vi "eMbot_EMG_viewer fun with shift registers.vi"() -> ()   [LabVIEW 2011]
uses:
  <vilib>/Utility/file.llb/Read From Spreadsheet File (DBL).vi
  <vilib>/Analysis/3filter.llb/Butterworth Filter (DBL).vi
  <vilib>/Analysis/1siggen.llb/Ramp Pattern by Samples.vi
  <vilib>/Analysis/8numeric.llb/1D Numeric Integration.vi
  <vilib>/Utility/file.llb/Write To Spreadsheet File (string).vi
  <vilib>/Analysis/NI_AALBase.lvlib
  <vilib>/Analysis/NI_AAL_SigProc.lvlib
  <vilib>/Analysis/NI_AALPro.lvlib
panel:
  in  "Use MVC?":bool
  in  "Data to Read":i32=-1
  in  "Side":u16(ring) items=["Right", "Left"]
  in  "Cycle-by-Cycle":bool=TRUE
  in  "Averaged Bins":bool=TRUE
  in  "Ensemble Averages":bool=TRUE
  in  "Select Muscles to Save":i32[](listbox)=[0, 1, 2, 3, 4, 5, 6, 7]
  in  "Save":bool
  in  "low cutoff freq":dbl=2.0
  in  "high cutoff freq":dbl=10.0
  in  "sampling freq":dbl=1000.0
  in  "Max EMG File":string="MVC1.txt"
  in  "Data Directory":string="C:\\Users\\PM&R\\Desktop\\Desktop Items\\Peter\\Data\\eMbot Testing Data\\"
  in  "Window Size":i32=10
  in  "peaks/valleys":enum32{"Peaks", "Valleys"}(ring)
  in  "Save Folder Name":string="EMG Postprocess"
  in  "Gait Event Channel":i32=18
  out "Locations":dbl[](array[numeric])
  in  "Stop":bool
  out "EMG Max":dbl
  in  "Threshold %Max":dbl=0.5
  in  "Shift Ensemble":i32
  out "RAW EMG":dbl[](graph)
  in  "Subject ID":string
  in  "Trial":i32
  out "Ensemble Average SD":dbl[](graph)
  out "Maximum EMG":dbl[](graph)
  out "Gait Event detection":cluster{"Ramp Pattern":dbl[], dbl[]}[](graph)
  in  "Muscle":i32
  out "Ensemble Average EMG":dbl[](graph)
  out "Spectrum Plot":cluster{dbl, "df":dbl, dbl[]}(graph)={0.0, "df"=0.5, []}
  out "Linear Envelope  EMG":dbl[](graph)
  out "Raw Gait Event Detection":dbl[](graph)
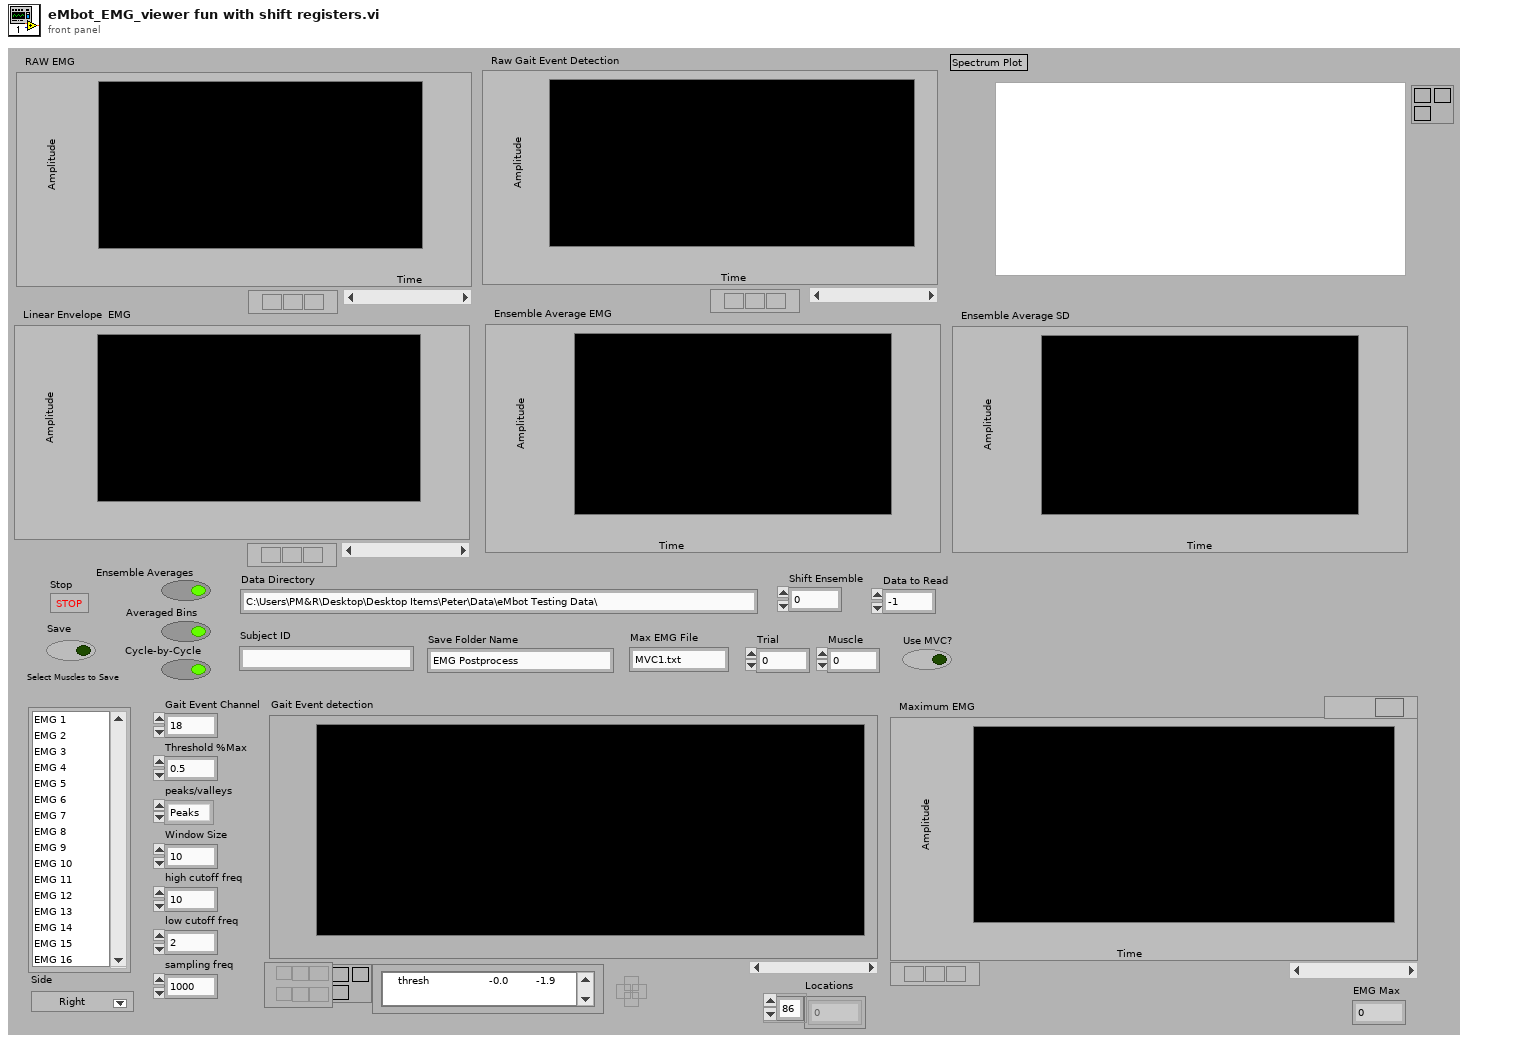
[diagram p1: front panel]
types:
  T1 = enum32{"Trapezoidal Rule", "Simpson's Rule", "Simpson's 3/8 Rule", "Bode Rule"}
  T2 = enum32{"Lowpass", "Highpass", "Bandpass", "Bandstop"}
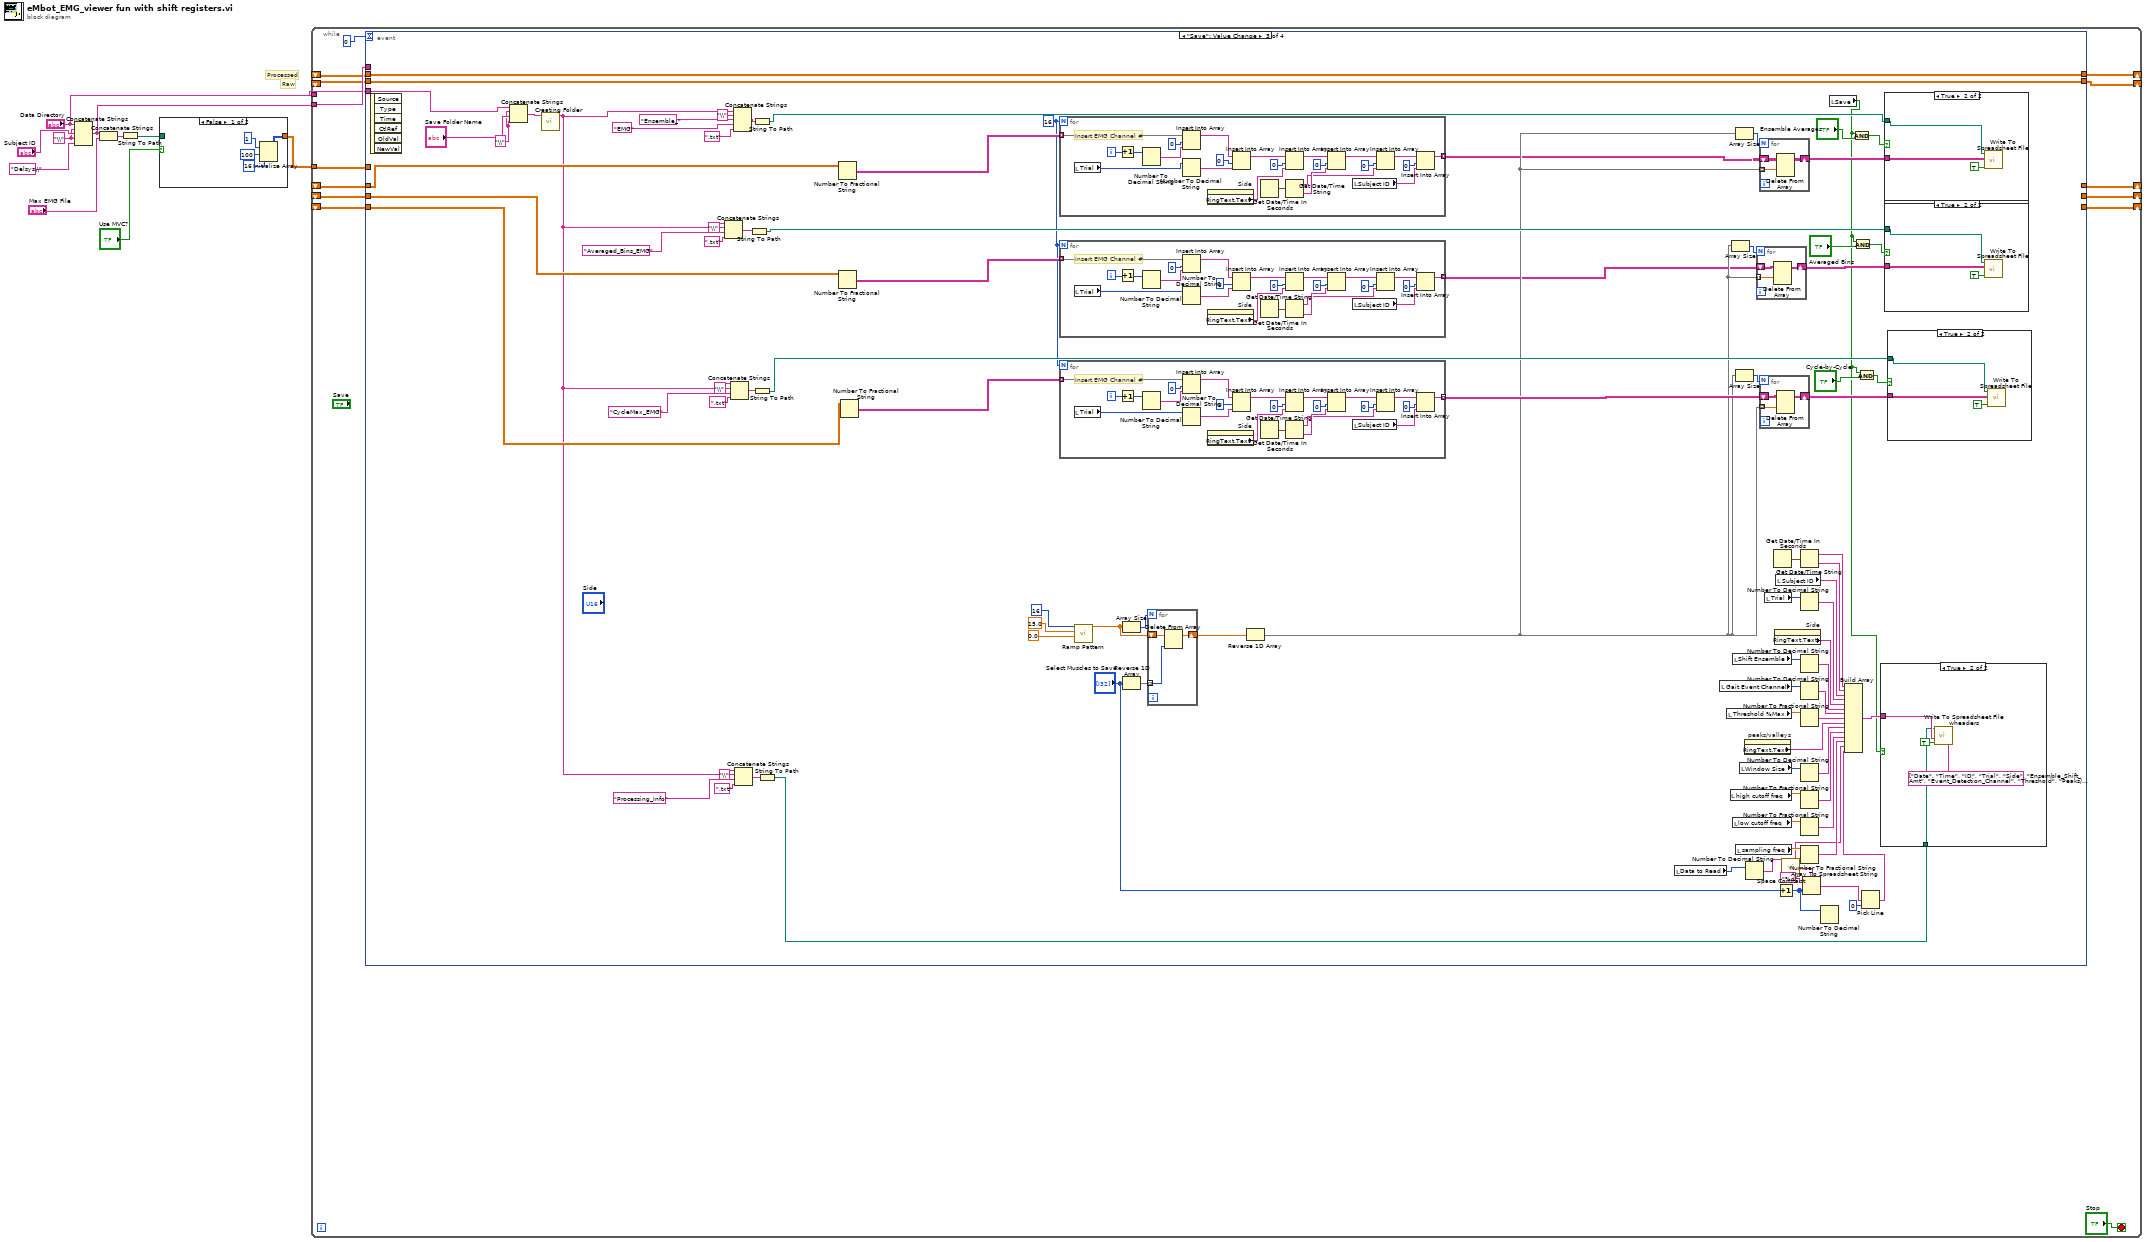
[diagram p0: block diagram]
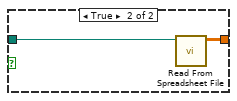
[diagram p2: hidden frame]
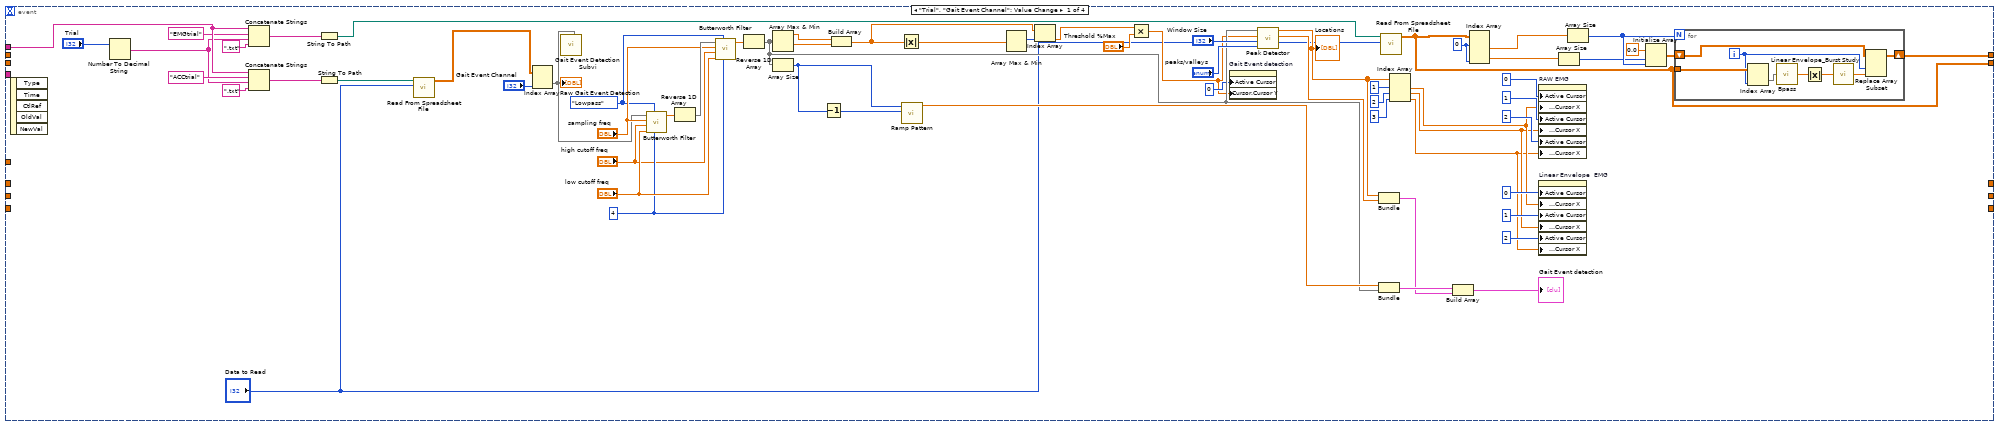
[diagram p3: hidden frame]
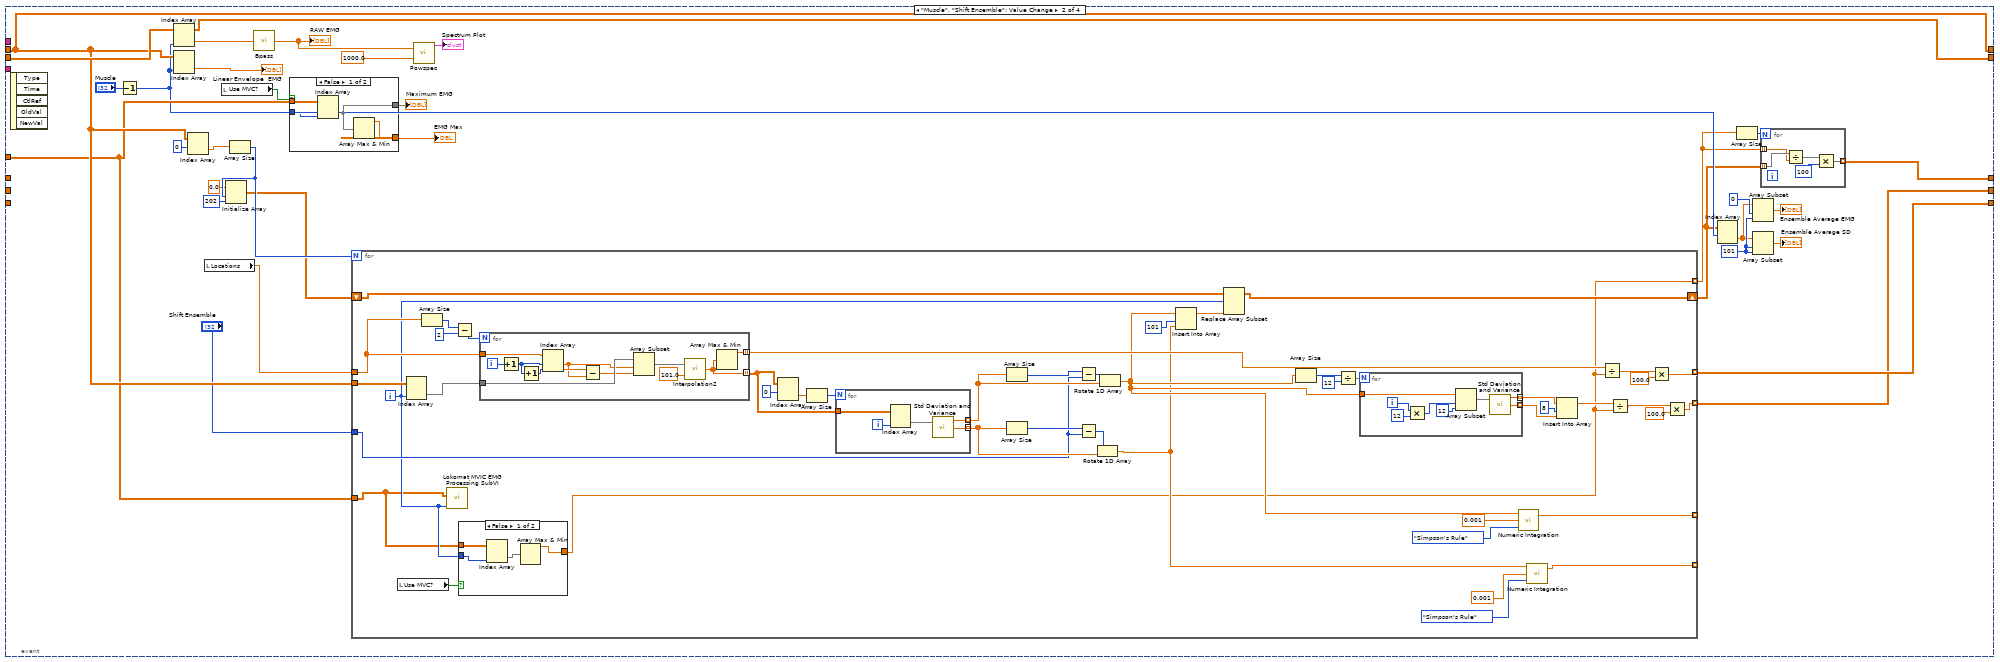
[diagram p4: hidden frame]
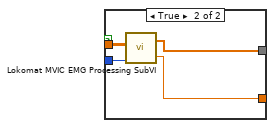
[diagram p5: hidden frame]
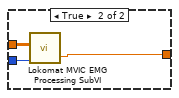
[diagram p6: hidden frame]
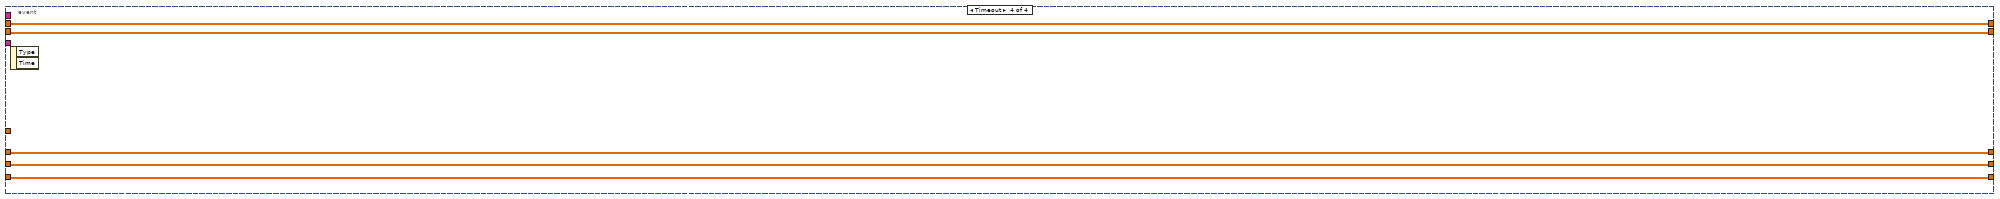
[diagram p11: hidden frame]
diagram:
  w3 = "\\" ("string")
  # "Raw"
  # "Processed"
  n1 = Concatenate Strings("Data Directory", w3, "Subject ID", w3, "Delsys\\" ("string")) -> (w5:string)
  n2 = Concatenate Strings(w5, "Max EMG File") -> (w8:string)
  n3 = String To Path(string=w8) -> (path=w9:path)
  n4 = case shown="False" "Use MVC?" {
    tunnel: w9 -> [_ w16]
    tunnel: [w13 w15] -> w4
    frame False {
      n5 = Initialize Array(1, 100 ("dimension size"), 16 ("dimension size")) -> (w13:i32[][])
    }
    frame True {
      n6 = call-poly <vilib>:"Read From Spreadsheet File.vi"("file path (dialog if empty)"=w16) -> ("all rows"=w15:dbl[][])  [unwired: 6 in, 4 out]
    }
  }
  n7 = while {
    tunnel: w5 -> [w30]
    tunnel: w4 -> [w28]
    shift-right: [w27] -> _
    shift-left: _ -> [w26]
    shift-right: [w25] -> _
    shift-left: _ -> [w24]
    shift-right: [w23] -> _
    shift-left: _ -> [w22]
    shift-right: [w21] -> _
    shift-left: _ -> [w20]
    shift-right: [w19] -> _
    shift-left: _ -> [w18]
    tunnel: "Data Directory" -> [w17]
    stop <- "Stop" stop-if-true
    n8 = event shown="[2] \"Save\": Value Change" {
      selector: _ -> [_ _ _ _]
      dyn-events: _ -> [_ _ _ _]
      timeout: 0 -> [_ _ _ _]
      tunnel: w30 -> [w62 _ _ _]
      tunnel: w28 -> [_ w114 _ _]
      tunnel: [_ w131 _ w413] -> w19
      tunnel: [w39 w126 w318 w417] -> w27
      tunnel: w26 -> [_ w126 w318 w417]
      tunnel: [w40 w127 w317 w416] -> w25
      tunnel: w24 -> [_ w127 w317 w416]
      tunnel: [_ w107 _ w415] -> w23
      tunnel: w22 -> [_ _ w305 w415]
      tunnel: [_ w106 _ w414] -> w21
      tunnel: w20 -> [_ _ w301 w414]
      tunnel: w18 -> [_ _ w293 w413]
      tunnel: w17 -> [_ _ w297 _]
      event "Trial", "Gait Event Channel": Value Change {
        w37 = 0 ("index (row)")
        w81 = T2."Lowpass" ("filter type")
        w82 = 4 ("order")
        n9 = event-data() -> ()  [unwired: 1 in, 5 out]
        n10 = Number To Decimal String(number="Trial") -> (decimal integer string=w56:string)  [unwired: 1 in]
        n11 = Concatenate Strings(w62, "EMGtrial" ("string"), w56, ".txt" ("string")) -> (w61:string)
        n12 = Concatenate Strings(w62, "ACCtrial" ("string"), w56, ".txt" ("string")) -> (w54:string)
        n13 = String To Path(string=w61) -> (path=w60:path)
        n14 = String To Path(string=w54) -> (path=w53:path)
        n15 = call-poly <vilib>:"Read From Spreadsheet File.vi"("number of rows (all:-1)"="Data to Read", "file path (dialog if empty)"=w53) -> ("all rows"=w95:dbl[][])  [unwired: 5 in, 4 out]
        n16 = Index Array(array=w95, index (col)="Gait Event Channel") -> (element=w50:dbl[])  [unwired: 1 in]
        "Raw Gait Event Detection" <- w50
        n17 = call "Gait Event Detection Subvi.vi"("Array"=w50) -> ()  [unwired: 1 in, 10 out]
        n18 = call-poly <vilib>:"Butterworth Filter.vi"("order"=w82, "filter type"=w81, "low cutoff freq: fl"="low cutoff freq", "high cutoff freq: fh"="high cutoff freq", "sampling freq: fs"="sampling freq", "X"=w50) -> ("Filtered X"=w87:dbl[])  [unwired: 2 in, 1 out]
        n19 = Reverse 1D Array(array=w87) -> (reversed array=w86:dbl[])
        n20 = call-poly <vilib>:"Butterworth Filter.vi"("order"=w82, "filter type"=w81, "low cutoff freq: fl"="low cutoff freq", "high cutoff freq: fh"="high cutoff freq", "sampling freq: fs"="sampling freq", "X"=w86) -> ("Filtered X"=w83:dbl[])  [unwired: 2 in, 1 out]
        n21 = Reverse 1D Array(array=w83) -> (reversed array=w64:dbl[])
        n22 = Array Max & Min(array=w64) -> (max value=w47:dbl, min value=w46:dbl)  [unwired: 2 out]
        n23 = Array Size(array=w64) -> (size(s)=w75:i32)
        n24 = Decrement(x=w75) -> (x-1=w76:i32)
        n25 = Build Array(w47, w46) -> (w43:dbl[])
        n26 = Absolute Value(x=w43) -> (abs(x)=w45:dbl[])
        n27 = call-poly <vilib>:"Ramp Pattern.vi"("end"=w76, "samples"=w75) -> ("Ramp Pattern"=w77:dbl[])  [unwired: 8 in, 1 out]
        n28 = Array Max & Min(array=w45) -> (max index (indices)=w42:i32)  [unwired: 3 out]
        n29 = Index Array(array=w43, index=w42) -> (element=w44:dbl)
        n30 = Multiply(x=w44, y="Threshold %Max") -> (x*y=w48:dbl)
        n31 = property on="Gait Event detection" class="XYGraph (strict)"("Active Cursor"=u32 0, "Cursor.Cursor Y"=w48) -> ()  [unwired: 2 in, 2 out]
        n32 = call <vilib>:"Peak Detector.vi"("peaks/valleys"="peaks/valleys", "width"="Window Size", "threshold"=w48, "X"=w64) -> ("Amplitudes"=w73:dbl[], "Locations"=w51:dbl[])  [unwired: 3 in, 3 out]
        "Locations" <- w51
        n33 = Bundle("Locations"=w51, "Amplitudes"=w73) -> (w72:cluster{"Locations":dbl[], "Amplitudes":dbl[]})  [unwired: 1 in]
        n34 = Bundle("Ramp Pattern"=w77, w64) -> (w74:cluster{"Ramp Pattern":dbl[], dbl[]})  [unwired: 1 in]
        n35 = call-poly <vilib>:"Read From Spreadsheet File.vi"("number of rows (all:-1)"="Data to Read", "file path (dialog if empty)"=w60) -> ("all rows"=w40:dbl[][])  [unwired: 5 in, 4 out]
        n36 = Index Array(array=w51, index #1=1 ("index"), index #2=2 ("index"), index #3=3 ("index")) -> (element #1=w67:dbl, element #2=w66:dbl, element #3=w65:dbl)
        n37 = Build Array(w74, w72) -> (→"Gait Event detection":cluster{"Locations":dbl[], "Amplitudes":dbl[]}[])
        n38 = Index Array(array=w40, index (row) #1=w37, index (col) #2=w37) -> (element #1=w41:dbl[], element #2=w36:dbl[])  [unwired: 2 in]
        n39 = property on="RAW EMG" class="WFGraph (strict)"("Active Cursor"=u32 0, "Cursor.Cursor Position:Cursor X"=w67, "Active Cursor"=u32 1, "Cursor.Cursor Position:Cursor X"=w66, "Active Cursor"=u32 2, "Cursor.Cursor Position:Cursor X"=w65) -> ()  [unwired: 2 in, 2 out]
        n40 = property on="Linear Envelope  EMG" class="WFGraph (strict)"("Active Cursor"=u32 0, "Cursor.Cursor Position:Cursor X"=w67, "Active Cursor"=u32 1, "Cursor.Cursor Position:Cursor X"=w66, "Active Cursor"=u32 2, "Cursor.Cursor Position:Cursor X"=w65) -> ()  [unwired: 2 in, 2 out]
        n41 = Array Size(array=w36) -> (size(s)=w35:i32)
        n42 = Array Size(array=w41) -> (size(s)=w38:i32)
        n43 = Initialize Array(0.0 ("element"), w35, w38) -> (w34:dbl[][])
        n44 = for {
          N: w38 -> [_]
          tunnel: w40 -> [w101]
          shift-right: [w96] -> w39
          shift-left: w34 -> [w98]
          i -> [w97]
          n45 = Index Array(array=w101, index (col)=w97) -> (element=w100:dbl[])  [unwired: 1 in]
          n46 = call "Bpass.vi"("Input Array"=w100) -> ("Output Array"=w102:dbl[])
          n47 = Absolute Value(x=w102) -> (abs(x)=w103:dbl[])
          n48 = call "Linear Envelope_Burst Study.vi"("Signals"=w103) -> ("Filtered Signals"=w99:dbl[])
          n49 = Replace Array Subset(array=w98, new element=w99, index (col)=w97) -> (w96:dbl[][])  [unwired: 1 in]
        }
      }
      event "Muscle", "Shift Ensemble": Value Change {
        w116 = 101 ("length")
        n50 = event-data() -> ()  [unwired: 1 in, 5 out]
        n51 = Decrement(x="Muscle") -> (x-1=w113:i32)
        n52 = Index Array(array=w127, index (col)=w113) -> (element=w130:dbl[])  [unwired: 1 in]
        n53 = Index Array(array=w126, index (col)=w113) -> (element=→"Linear Envelope  EMG":dbl[])  [unwired: 1 in]
        n54 = Index Array(array=w126, index (row)=0) -> (element=w124:dbl[])  [unwired: 1 in]
        n55 = local read "Locations"() -> (w132:dbl[])
        n56 = local read "Use MVC?"() -> (w104:bool)
        n57 = Array Size(array=w124) -> (size(s)=w123:i32)
        n58 = Initialize Array(0.0 ("element"), w123, 202 ("dimension size")) -> (w121:dbl[][])
        n59 = call "Bpass.vi"("Input Array"=w130) -> ("Output Array"=w129:dbl[])
        "RAW EMG" <- w129
        n60 = case shown="False" w104 {
          tunnel: w114 -> [w139 w143]
          tunnel: w113 -> [w138 w142]
          tunnel: [w137 w141] -> w112
          tunnel: [w136 w140] -> w111
          frame False {
            n61 = Index Array(array=w139, index (col)=w138) -> (element=w137:dbl[])  [unwired: 1 in]
            n62 = Array Max & Min(array=w137) -> (max value=w136:dbl)  [unwired: 3 out]
          }
          frame True {
            n63 = call "Lokomat MVIC EMG Processing SubVI.vi"("EMG Channel"=w142, "Input Array"=w143) -> ("EMG Max"=w140:dbl, "EMG"=w141:dbl[])  [unwired: 2 in]
          }
        }
        "Maximum EMG" <- w112
        "EMG Max" <- w111
        n64 = for {
          N: w123 -> [_]
          tunnel: w126 -> [w166]
          tunnel: w132 -> [w195]
          tunnel: [w172] -> w131 mode=indexing
          shift-right: [w158] -> w110
          shift-left: w121 -> [w161]
          tunnel: [w160] -> _ mode=indexing
          tunnel: [w159] -> _ mode=indexing
          tunnel: w114 -> [w150]
          tunnel: [w149] -> w108 mode=indexing
          tunnel: [w155] -> w106 mode=indexing
          tunnel: "Shift Ensemble" -> [w153]
          i -> [w151]
          n65 = local read "Use MVC?"() -> (w152:bool)
          n66 = Index Array(array=w166, index (col)=w151) -> (element=w165:dbl[])  [unwired: 1 in]
          n67 = Array Size(array=w195) -> (size(s)=w174:i32)
          n68 = call "Lokomat MVIC EMG Processing SubVI.vi"("EMG Channel"=w151, "Input Array"=w150) -> ()  [unwired: 2 in, 2 out]
          n69 = Subtract(x=w174, y=2) -> (x-y=w185:i32)
          n70 = case shown="False" w152 {
            tunnel: w150 -> [w199 w202]
            tunnel: w151 -> [w198 w201]
            tunnel: [w196 w200] -> w149
            frame False {
              n71 = Index Array(array=w199, index (col)=w198) -> (element=w197:dbl[])  [unwired: 1 in]
              n72 = Array Max & Min(array=w197) -> (max value=w196:dbl)  [unwired: 3 out]
            }
            frame True {
              n73 = call "Lokomat MVIC EMG Processing SubVI.vi"("EMG Channel"=w201, "Input Array"=w202) -> ("EMG Max"=w200:dbl)  [unwired: 2 in, 1 out]
            }
          }
          n74 = for {
            N: w185 -> [_]
            tunnel: w165 -> [w227]
            tunnel: w195 -> [w225]
            tunnel: [w217] -> w167 mode=indexing
            tunnel: [w216] -> w194 mode=indexing
            i -> [w226]
            n75 = Increment(x=w226) -> (x+1=w224:i32)
            n76 = Increment(x=w224) -> (x+1=w223:i32)
            n77 = Index Array(array=w225, index #1=w224, index #2=w223) -> (element #1=w218:dbl, element #2=w222:dbl)
            n78 = Subtract(x=w222, y=w218) -> (x-y=w219:dbl)
            n79 = Array Subset(array=w227, index=w218, length=w219) -> (w221:dbl[])
            n80 = call "Interpolation2.vi"("Normalize to # of Data Points"=101.0, "Original Array"=w221) -> ("Normalized Array"=w217:dbl[])
            n81 = Array Max & Min(array=w217) -> (max value=w216:dbl)  [unwired: 3 out]
          }
          n82 = Index Array(array=w167, index (row)=0) -> (element=w177:dbl[])  [unwired: 1 in]
          n83 = Array Size(array=w177) -> (size(s)=w178:i32)
          n84 = for {
            N: w178 -> [_]
            tunnel: w167 -> [w215]
            tunnel: [w212] -> w188 mode=indexing
            tunnel: [w211] -> w191 mode=indexing
            i -> [w214]
            n85 = Index Array(array=w215, index (col)=w214) -> (element=w213:dbl[])  [unwired: 1 in]
            n86 = call <vilib>:"Std Deviation and Variance.vi"("X"=w213) -> ("mean"=w212:dbl, "standard deviation"=w211:dbl)  [unwired: 1 in, 1 out]
          }
          n87 = Array Size(array=w188) -> (size(s)=w186:i32)
          n88 = Array Size(array=w191) -> (size(s)=w189:i32)
          n89 = Subtract(x=w186, y=w153) -> (x-y=w187:i32)
          n90 = Subtract(x=w189, y=w153) -> (x-y=w190:i32)
          n91 = Rotate 1D Array(1:w191, 2:w190) -> (0:w163:dbl[])
          n92 = Rotate 1D Array(1:w188, 2:w187) -> (0:w164:dbl[])
          n93 = Insert Into Array(array=w164, index=101, new element=w163) -> (w162:dbl[])
          n94 = Replace Array Subset(array=w161, new element=w162, index (row)=w151) -> (w158:dbl[][])  [unwired: 1 in]
          n95 = Array Size(array=w164) -> (size(s)=w180:i32)
          n96 = Divide(x=w180, y=12) -> (x/y=w179:dbl)
          n97 = for {
            N: w179 -> [_]
            tunnel: w164 -> [w210]
            tunnel: [w204] -> w182 mode=indexing
            tunnel: [w203] -> w184 mode=indexing
            i -> [w209]
            n98 = Multiply(x=w209, y=12) -> (x*y=w207:i32)
            n99 = Array Subset(array=w210, index=w207, length=12) -> (w205:dbl[])
            n100 = call <vilib>:"Std Deviation and Variance.vi"("X"=w205) -> ("mean"=w204:dbl, "standard deviation"=w203:dbl)  [unwired: 1 in, 1 out]
          }
          n101 = call-poly <vilib>:"Numeric Integration.vi"("integration method"=T1."Simpson's Rule", "dt"=0.001, "Input Array"=w164) -> ("result"=w160:dbl)  [unwired: 1 out]
          n102 = call-poly <vilib>:"Numeric Integration.vi"("integration method"=T1."Simpson's Rule", "dt"=0.001, "Input Array"=w163) -> ("result"=w159:dbl)  [unwired: 1 out]
          n103 = Insert Into Array(array=w182, index=8, new element=w184) -> (w157:dbl[])
          n104 = Divide(x=w194, y=w149) -> (x/y=w192:dbl[])
          n105 = Divide(x=w157, y=w149) -> (x/y=w154:dbl[])
          n106 = Multiply(x=w192, y=100.0) -> (x*y=w172:dbl[])
          n107 = Multiply(x=w154, y=100.0) -> (x*y=w155:dbl[])
        }
        n108 = call "Powspec.vi"("Emg input"=w129, "Sample rate"=sgl 1000.0) -> ("Spectrum Plot"=→"Spectrum Plot":cluster{dbl, "df":dbl, dbl[]})  [unwired: 5 out]
        n109 = Index Array(array=w110, index (row)=w113) -> (element=w115:dbl[])  [unwired: 1 in]
        n110 = Array Size(array=w108) -> (size(s)=w109:i32)
        n111 = Array Subset(array=w115, index=0, length=w116) -> (→"Ensemble Average EMG":dbl[])
        n112 = Array Subset(array=w115, index=w116, length=w116) -> (→"Ensemble Average SD":dbl[])
        n113 = for {
          N: w109 -> [_]
          tunnel: w108 -> [w147] mode=indexing
          tunnel: w110 -> [w148] mode=indexing
          tunnel: [w144] -> w107 mode=indexing
          n114 = Divide(x=w148, y=w147) -> (x/y=w146:dbl[])
          n115 = Multiply(x=w146, y=100) -> (x*y=w144:dbl[])
        }
      }
      event "Save": Value Change {
        w231 = 16
        w298 = "\\" ("string")
        n116 = event-data() -> ()  [unwired: 1 in, 6 out]
        n117 = Concatenate Strings(w297, w298, "Save Folder Name", w298) -> (w316:string)
        n118 = call "Creating Folder.vi"("Input String Path"=w316) -> ("Output String Path"=w254:string)  [unwired: 10 in]
        n119 = Concatenate Strings(w254, "\\" ("string"), "Averaged_Bins_EMG", ".txt" ("string")) -> (w308:string)
        n120 = Concatenate Strings(w254, "\\" ("string"), "CycleMax_EMG", ".txt" ("string")) -> (w313:string)
        n121 = Concatenate Strings(w254, "\\" ("string"), "Ensemble_" ("string"), "EMG", ".txt" ("string")) -> (w310:string)
        n122 = Concatenate Strings(w254, "\\" ("string"), "Processing_Info", ".txt" ("string")) -> (w256:string)
        n123 = String To Path(string=w308) -> (path=w302:path)
        n124 = String To Path(string=w310) -> (path=w306:path)
        n125 = String To Path(string=w313) -> (path=w299:path)
        n126 = String To Path(string=w256) -> (path=w253:path)
        n127 = Number To Fractional String(number=w305) -> (F-format string=w245:string[][])  [unwired: 3 in]
        n128 = Number To Fractional String(number=w301) -> (F-format string=w247:string[][])  [unwired: 3 in]
        n129 = Number To Fractional String(number=w293) -> (F-format string=w300:string[][])  [unwired: 3 in]
        n130 = for {
          N: w231 -> [_]
          tunnel: w245 -> [w343] mode=indexing
          tunnel: [w340] -> w244 mode=indexing
          i -> [w335]
          # "Insert EMG Channel #"
          n131 = local read "Trial"() -> (w336:i32)
          n132 = Increment(x=w335) -> (x+1=w334:i32)
          n133 = Number To Decimal String(number=w334) -> (decimal integer string=w342:string)  [unwired: 1 in]
          n134 = Insert Into Array(array=w343, index=0, new element=w342) -> (w339:string[])
          n135 = Number To Decimal String(number=w336) -> (decimal integer string=w337:string)  [unwired: 1 in]
          n136 = property on="Side" class="Ring (strict)"() -> ("RingText.Text"=w332:string)  [unwired: 2 in, 2 out]
          n137 = Insert Into Array(array=w339, index=0, new element=w337) -> (w331:string[])
          n138 = Get Date/Time In Seconds() -> (seconds since 1Jan1904=w330:timestamp)
          n139 = Insert Into Array(array=w331, index=0, new element=w332) -> (w328:string[])
          n140 = Get Date/Time String(seconds (now)=w330) -> (date string=w323:string, time string=w324:string)  [unwired: 2 in]
          n141 = Insert Into Array(array=w328, index=0, new element=w324) -> (w329:string[])
          n142 = local read "Subject ID"() -> (w341:string)
          n143 = Insert Into Array(array=w329, index=0, new element=w323) -> (w327:string[])
          n144 = Insert Into Array(array=w327, index=0, new element=w341) -> (w340:string[])
        }
        n145 = for {
          N: w231 -> [_]
          tunnel: w247 -> [w366] mode=indexing
          tunnel: [w363] -> w246 mode=indexing
          i -> [w358]
          # "Insert EMG Channel #"
          n146 = local read "Trial"() -> (w359:i32)
          n147 = Increment(x=w358) -> (x+1=w357:i32)
          n148 = Number To Decimal String(number=w357) -> (decimal integer string=w365:string)  [unwired: 1 in]
          n149 = Insert Into Array(array=w366, index=0, new element=w365) -> (w362:string[])
          n150 = Number To Decimal String(number=w359) -> (decimal integer string=w360:string)  [unwired: 1 in]
          n151 = property on="Side" class="Ring (strict)"() -> ("RingText.Text"=w355:string)  [unwired: 2 in, 2 out]
          n152 = Insert Into Array(array=w362, index=0, new element=w360) -> (w354:string[])
          n153 = Get Date/Time In Seconds() -> (seconds since 1Jan1904=w353:timestamp)
          n154 = Insert Into Array(array=w354, index=0, new element=w355) -> (w351:string[])
          n155 = Get Date/Time String(seconds (now)=w353) -> (date string=w346:string, time string=w347:string)  [unwired: 2 in]
          n156 = Insert Into Array(array=w351, index=0, new element=w347) -> (w352:string[])
          n157 = local read "Subject ID"() -> (w364:string)
          n158 = Insert Into Array(array=w352, index=0, new element=w346) -> (w350:string[])
          n159 = Insert Into Array(array=w350, index=0, new element=w364) -> (w363:string[])
        }
        n160 = for {
          N: w231 -> [_]
          tunnel: w300 -> [w401] mode=indexing
          tunnel: [w398] -> w291 mode=indexing
          i -> [w393]
          # "Insert EMG Channel #"
          n161 = local read "Trial"() -> (w394:i32)
          n162 = Increment(x=w393) -> (x+1=w392:i32)
          n163 = Number To Decimal String(number=w392) -> (decimal integer string=w400:string)  [unwired: 1 in]
          n164 = Insert Into Array(array=w401, index=0, new element=w400) -> (w397:string[])
          n165 = Number To Decimal String(number=w394) -> (decimal integer string=w395:string)  [unwired: 1 in]
          n166 = property on="Side" class="Ring (strict)"() -> ("RingText.Text"=w390:string)  [unwired: 2 in, 2 out]
          n167 = Insert Into Array(array=w397, index=0, new element=w395) -> (w389:string[])
          n168 = Get Date/Time In Seconds() -> (seconds since 1Jan1904=w388:timestamp)
          n169 = Insert Into Array(array=w389, index=0, new element=w390) -> (w386:string[])
          n170 = Get Date/Time String(seconds (now)=w388) -> (date string=w381:string, time string=w382:string)  [unwired: 2 in]
          n171 = Insert Into Array(array=w386, index=0, new element=w382) -> (w387:string[])
          n172 = local read "Subject ID"() -> (w399:string)
          n173 = Insert Into Array(array=w387, index=0, new element=w381) -> (w385:string[])
          n174 = Insert Into Array(array=w385, index=0, new element=w399) -> (w398:string[])
        }
        n175 = call-poly <vilib>:"Ramp Pattern.vi"("start"=0.0, "end"=15.0, "samples"=16) -> ("Ramp Pattern"=w285:dbl[])  [unwired: 7 in, 1 out]
        n176 = Array Size(array=w285) -> (size(s)=w287:i32)
        n177 = Reverse 1D Array(array="Select Muscles to Save") -> (reversed array=w286:i32[])
        n178 = for {
          N: w287 -> [_]
          tunnel: w286 -> [w379] mode=indexing
          shift-right: [w378] -> w273
          shift-left: w285 -> [w380]
          n179 = Delete From Array(array=w380, index=w379) -> (array with subset deleted=w378:dbl[])  [unwired: 1 in, 1 out]
        }
        n180 = Reverse 1D Array(array=w273) -> (reversed array=w280:dbl[])
        n181 = local read "Data to Read"() -> (w229:i32)
        n182 = local read "Gait Event Channel"() -> (w269:i32)
        n183 = local read "Threshold %Max"() -> (w268:dbl)
        n184 = local read "high cutoff freq"() -> (w266:dbl)
        n185 = Array Size(array=w280) -> (size(s)=w283:i32)
        n186 = local read "Shift Ensemble"() -> (w272:i32)
        n187 = local read "low cutoff freq"() -> (w265:dbl)
        n188 = Array Size(array=w280) -> (size(s)=w281:i32)
        n189 = Array Size(array=w280) -> (size(s)=w292:i32)
        n190 = local read "sampling freq"() -> (w264:dbl)
        n191 = local read "Window Size"() -> (w267:i32)
        n192 = property on="peaks/valleys" class="Enum (strict)"() -> ("RingText.Text"=w243:string)  [unwired: 2 in, 2 out]
        n193 = Number To Decimal String(number=w229) -> (decimal integer string=w228:string)  [unwired: 1 in]
        n194 = for {
          N: w283 -> [_]
          tunnel: w280 -> [w373] mode=indexing
          shift-right: [w372] -> w282
          shift-left: w246 -> [w374]
          n195 = Delete From Array(array=w374, index (row)=w373) -> (array with subset deleted=w372:string[][])  [unwired: 2 in, 1 out]
        }
        n196 = for {
          N: w281 -> [_]
          tunnel: w280 -> [w370] mode=indexing
          shift-right: [w369] -> w279
          shift-left: w244 -> [w371]
          n197 = Delete From Array(array=w371, index (row)=w370) -> (array with subset deleted=w369:string[][])  [unwired: 2 in, 1 out]
        }
        n198 = for {
          N: w292 -> [_]
          tunnel: w280 -> [w376] mode=indexing
          shift-right: [w375] -> w284
          shift-left: w291 -> [w377]
          n199 = Delete From Array(array=w377, index (row)=w376) -> (array with subset deleted=w375:string[][])  [unwired: 2 in, 1 out]
        }
        n200 = local read "Trial"() -> (w277:i32)
        n201 = Get Date/Time In Seconds() -> (seconds since 1Jan1904=w262:timestamp)
        n202 = property on="Side" class="Ring (strict)"() -> ("RingText.Text"=w275:string)  [unwired: 2 in, 2 out]
        n203 = local read "Subject ID"() -> (w278:string)
        n204 = Increment(x="Select Muscles to Save") -> (x+1=w241:i32[])
        n205 = call <vilib>:"Space Constant.vi"() -> ("String"=w242:string)
        n206 = Get Date/Time String(seconds (now)=w262) -> (date string=w261:string, time string=w260:string)  [unwired: 2 in]
        n207 = Number To Decimal String(number=w277) -> (decimal integer string=w276:string)  [unwired: 1 in]
        n208 = Number To Decimal String(number=w272) -> (decimal integer string=w271:string)  [unwired: 1 in]
        n209 = Number To Decimal String(number=w269) -> (decimal integer string=w270:string)  [unwired: 1 in]
        n210 = Number To Fractional String(number=w268) -> (F-format string=w252:string)  [unwired: 3 in]
        n211 = Number To Decimal String(number=w267) -> (decimal integer string=w251:string)  [unwired: 1 in]
        n212 = Number To Fractional String(number=w266) -> (F-format string=w250:string)  [unwired: 3 in]
        n213 = Number To Fractional String(number=w265) -> (F-format string=w249:string)  [unwired: 3 in]
        n214 = Number To Fractional String(number=w264) -> (F-format string=w248:string)  [unwired: 3 in]
        n215 = Array To Spreadsheet String(delimiter (Tab)=w242, array=w241, 3:"%d" ("format string")) -> (spreadsheet string=w239:string)
        n216 = Number To Decimal String(number=w241) -> ()  [unwired: 1 in, 1 out]
        n217 = local read "Save"() -> (w232:bool)
        n218 = And(x=w232, y="Ensemble Averages") -> (x .and. y?=w237:bool)
        n219 = And(x=w232, y="Averaged Bins") -> (x .and. y?=w233:bool)
        n220 = And(x=w232, y="Cycle-by-Cycle") -> (x .and. y?=w235:bool)
        n221 = Pick Line(multi-line string=w239, line index=0) -> (output string=w230:string)  [unwired: 1 in]
        n222 = Build Array(w261, w260, w278, w276, w275, w271, w270, w252, w243, w251, w250, w249, w248, w228, w230) -> (w259:string[])
        n223 = case shown="True" w232 {
          tunnel: w259 -> [_ w322]
          tunnel: w253 -> [_ w321]
          frame False {
          }
          frame True {
            n224 = call "Write To Spreadsheet File wheaders.vi"("Headers"=string[] ["Date", "Time", "ID", "Trial", "Side", "Ensemble_Shift_Amt", "Event_Detection_Channel", "Threshold", "Peaks/Valleys", "Window_Size", "Highpass_Cutoff", "Lowpass_Cutoff", "Sampling_Freq", "Saved Channels"], "append to file? (new file:F)"=TRUE, "1D data"=w322, "file path (dialog if empty)"=w321) -> ()  [unwired: 4 in, 1 out]
          }
        }
        n225 = case shown="True" w237 {
          tunnel: w306 -> [_ w412]
          tunnel: w279 -> [_ w411]
          frame False {
          }
          frame True {
            n226 = call-poly <vilib>:"Write To Spreadsheet File.vi"("append to file? (new file:F)"=TRUE, "2D data"=w411, "file path (dialog if empty)"=w412) -> ()  [unwired: 5 in, 1 out]
          }
        }
        n227 = case shown="True" w233 {
          tunnel: w302 -> [_ w409]
          tunnel: w282 -> [_ w408]
          frame False {
          }
          frame True {
            n228 = call-poly <vilib>:"Write To Spreadsheet File.vi"("append to file? (new file:F)"=TRUE, "2D data"=w408, "file path (dialog if empty)"=w409) -> ()  [unwired: 5 in, 1 out]
          }
        }
        n229 = case shown="True" w235 {
          tunnel: w299 -> [_ w406]
          tunnel: w284 -> [_ w405]
          frame False {
          }
          frame True {
            n230 = call-poly <vilib>:"Write To Spreadsheet File.vi"("append to file? (new file:F)"=TRUE, "2D data"=w405, "file path (dialog if empty)"=w406) -> ()  [unwired: 5 in, 1 out]
          }
        }
      }
      event Timeout {
        n231 = event-data() -> ()  [unwired: 1 in, 2 out]
      }
    }
  }
